vi "acquisition.vi"(8 "error in (no error)":errorcluster, 11 "DAQCascade512II":refnum<class "DAQCascade512II.lvclass">) -> (0 "error out":errorcluster, 3 "DAQCascade512II out":refnum<class "DAQCascade512II.lvclass">)   [LabVIEW 2012, in "DAQCascade512II.lvclass"]
uses:
  DAQCascade512II.lvclass
  DAQCascade512II.lvclass/DAQCascade512II.ctl
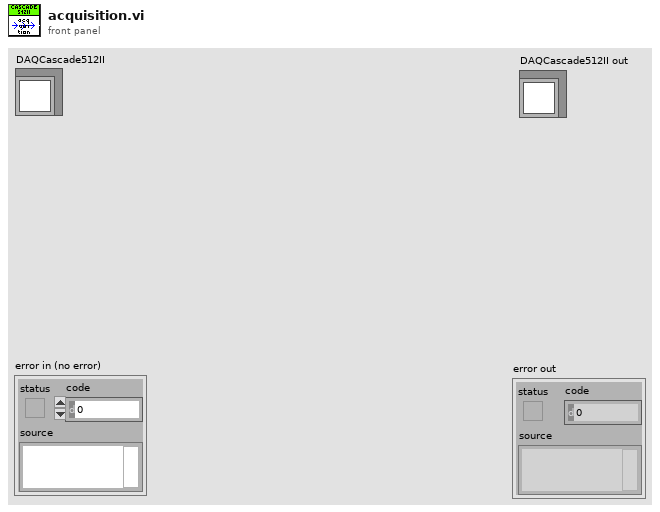
[diagram p1: front panel]
types:
  T1 = cluster{"Array uint 16":u16[][], "setting.File Path":path}
  T2 = typedef "DAQCascade512II.lvclass/File Path.ctl" = path
  T3 = typedef "IMAQ Image.ctl" = refnum<image>
  T4 = typedef "DAQCascade512II.lvclass/focus or acquire.ctl" = bool
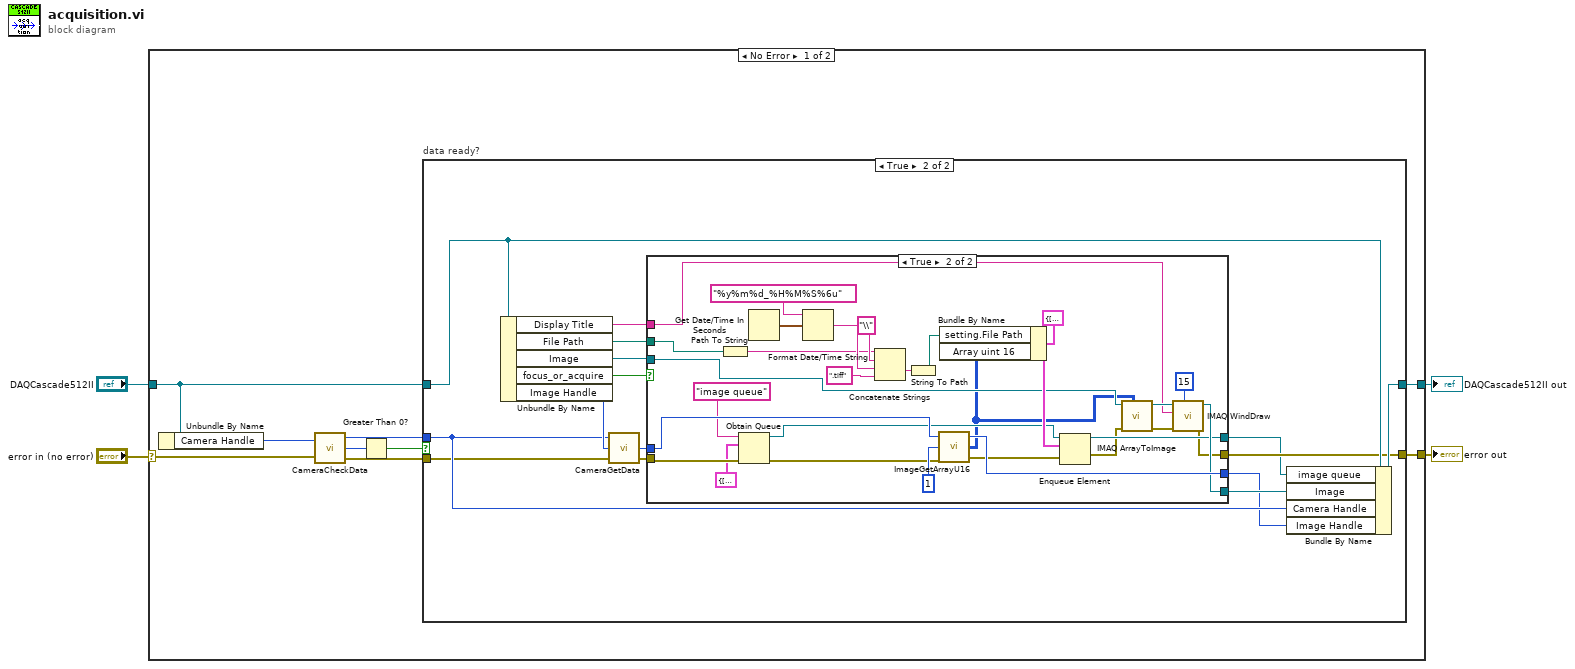
[diagram p0: block diagram]
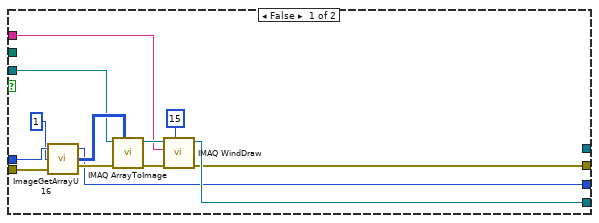
[diagram p3: hidden frame]
diagram:
  n1 = case shown="No Error" "error in (no error)" {
    selector: "error in (no error)" -> [w5 w75]
    tunnel: [w13 w74] -> w4
    tunnel: [w12 w75] -> w3
    tunnel: "DAQCascade512II" -> [w11 w74]
    frame No Error {
      n2 = Unbundle By Name(w11) -> ("Camera Handle"=w10:u32)
      n3 = call <userlib>:"CameraCheckData.vi"("Camera Handle"=w10, "error in"=w5) -> ("Camera Handle"=w7:u32, "Number Of Frames Available"=w9:i32, "error out"=w6:errorcluster)
      n4 = Greater Than 0?(x=w9) -> (x > 0?=w8:bool)
      n5 = case "data ready?" shown="True" w8 {
        tunnel: w7 -> [_ w24]
        tunnel: w11 -> [w15 w30]
        tunnel: w6 -> [w14 w23]
        tunnel: [w15 w29] -> w13
        tunnel: [w14 w28] -> w12
        frame False {
        }
        frame True {
          n6 = Unbundle By Name(w30) -> ("Display Title"=w16:string, "File Path"=w17:T2, "Image"=w19:T3, "focus_or_acquire"=w27:T4, "Image Handle"=w25:u32)
          n7 = call <userlib>:"CameraGetData.vi"("error in"=w23, "Data Handle"=w25, "Camera Handle"=w24) -> ("error out"=w22:errorcluster, "Data Handle"=w21:u32)  [unwired: 1 out]
          n8 = case shown="True" w27 {
            tunnel: w22 -> [w40 w57]
            tunnel: [w41 w44] -> w28
            tunnel: [w42 w47] -> w26
            tunnel: w21 -> [w39 w73]
            tunnel: [w33 w72] -> w20
            tunnel: w19 -> [w32 w50]
            tunnel: [_ w46] -> w18
            tunnel: w17 -> [_ w61]
            tunnel: w16 -> [w31 w49]
            frame False {
              n9 = call <userlib>:"ImageGetArrayU16.vi"("error in"=w40, "Z position"=u32 1, "Image Handle"=w39) -> ("error out"=w36:errorcluster, "Array uint 16"=w37:u16[][], "Image Handle"=w33:u32)
              n10 = call "IMAQ ArrayToImage"("Image Pixels (U16)"=w37, "error in (no error)"=w36, "Image"=w32) -> ("error out"=w35:errorcluster, "Image Out"=w34:T3)  [unwired: 7 in]
              n11 = call "IMAQ WindDraw"("Window Number (0...15)"=15, "error in (no error)"=w35, "Title"=w31, "Image"=w34) -> ("error out"=w41:errorcluster, "Image Out (duplicate)"=w42:T3)  [unwired: 6 in]
            }
            frame True {
              n12 = Path To String(path=w61) -> (string=w59:string)
              n13 = Obtain Queue(name (unnamed)="image queue", element data type=T1 {"Array uint 16"=[], "setting.File Path"=path ""}, error in (no error)=w57) -> (queue out=w56:refnum<queue>, error out=w55:errorcluster)  [unwired: 2 in, 1 out]
              n14 = Get Date/Time In Seconds() -> (seconds since 1Jan1904=w66:timestamp)
              n15 = Format Date/Time String(time format string (%c)="%y%m%d_%H%M%S%6u", seconds (now)=w66) -> (date/time string=w64:string)  [unwired: 1 in]
              n16 = Concatenate Strings(w59, "\\" ("string"), w64, ".tiff" ("string")) -> (w62:string)
              n17 = String To Path(string=w62) -> (path=w60:path)
              n18 = call <userlib>:"ImageGetArrayU16.vi"("error in"=w55, "Z position"=u32 1, "Image Handle"=w73) -> ("error out"=w68:errorcluster, "Array uint 16"=w48:u16[][], "Image Handle"=w72:u32)
              n19 = Bundle By Name(cluster=T1 {"Array uint 16"=[], "setting.File Path"=path ""}, "setting.File Path"=w60, "Array uint 16"=w48) -> (w69:T1)
              n20 = Enqueue Element(queue=w56, element=w69, error in (no error)=w68) -> (queue out=w46:refnum<queue>, error out=w45:errorcluster)  [unwired: 1 in, 1 out]
              n21 = call "IMAQ ArrayToImage"("Image Pixels (U16)"=w48, "error in (no error)"=w45, "Image"=w50) -> ("error out"=w52:errorcluster, "Image Out"=w51:T3)  [unwired: 7 in]
              n22 = call "IMAQ WindDraw"("Window Number (0...15)"=15, "error in (no error)"=w52, "Title"=w49, "Image"=w51) -> ("error out"=w44:errorcluster, "Image Out (duplicate)"=w47:T3)  [unwired: 6 in]
            }
          }
          n23 = Bundle By Name(cluster=w30, "image queue"=w18, "Image"=w26, "Camera Handle"=w24, "Image Handle"=w20) -> (w29:refnum<class "DAQCascade512II.lvclass">)
        }
      }
    }
    frame Error {
    }
  }
  "error out" <- w3
  "DAQCascade512II out" <- w4
